vi "Is Marked For Destroy.vi"(11 "Actor in":refnum<class "Actor.lvclass">) -> (2 "Is Marked For Destroy":bool)   [LabVIEW 2020, in "jettl.lvlib" / "Actor.lvlib" / "Actor.lvclass"]
uses:
  Actor.lvclass
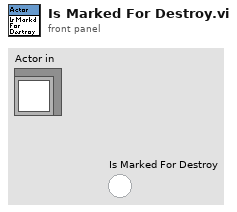
[diagram p1: front panel]
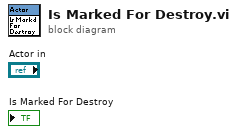
[diagram p0: block diagram]
diagram:
